vi "界面UI.vi"() -> ()   [LabVIEW 2016, in "科盛超标留样.lvlib"]
uses:
  <vilib>/Utility/miscctls.llb/LVPointTypeDef.ctl
  <vilib>/Utility/config.llb/NI_LVConfig.lvlib
  <vilib>/ptbypt/NI_PtbyPt.lvlib
panel:
  in  "超标浓度配置":bool
  in  "清除瓶记录":bool
  in  "停止流程":bool
  in  "启动流程":bool
  out "流程中":bool
  out "留样等待时间/s":dbl
  out "供样等待时间/s":dbl
  out "采样等待时间/s":dbl
  out "留样完成":bool
  out "采样完成":bool
  out "开关量3状态":T1
  out "开关量2状态":T2
  out "开关量1状态":T3
  out "元素":enum16{"open", "read", "write", "close"}(ring)
  out "供样完成":bool
  in  "返回":bool
  in  "查看记录":bool
  in  "当前解析模式":string(combo)
  in  "切换串口":bool
  out "查询系统状态":T4
  out "查询瓶记录":T5
  out "输出数组":T6(array[cluster])
  in  "留样命令":bool
  in  "供样命令":bool
  in  "触发采样":bool
  in  "查询系统状态":bool
  in  "远程取样":bool
  in  "复位指令":bool
  in  "查询瓶记录":bool
  in  "查询采样记录":bool
  in  "VISA resource name":refnum<visa-resource-name>="COM2" caption="VISA资源名称"
  in  "写入缓冲区":string
  out "读取缓冲区":string
  out "source":string
  out "通讯":bool
  # "启动顺序：先触发采样将水样取到A、B桶，然后仪器开始测试时发送供样命令此时供应到分析仪，如果超标发送留样命令，如果在默认60分钟(可设置)后都没有接受到超标留\n样指令则自动排空。按不同的采样方式发送不同的通信字符串。在一次采样未结束前不要发送下一个采样指令。"
  # "采样：将水样取到A、B桶的过程；\n供样：将水样从A、B桶供应到分析仪的过程；\n留样：将水样从A、B桶保存到采样瓶的过程。"
  # "科盛超标留样"
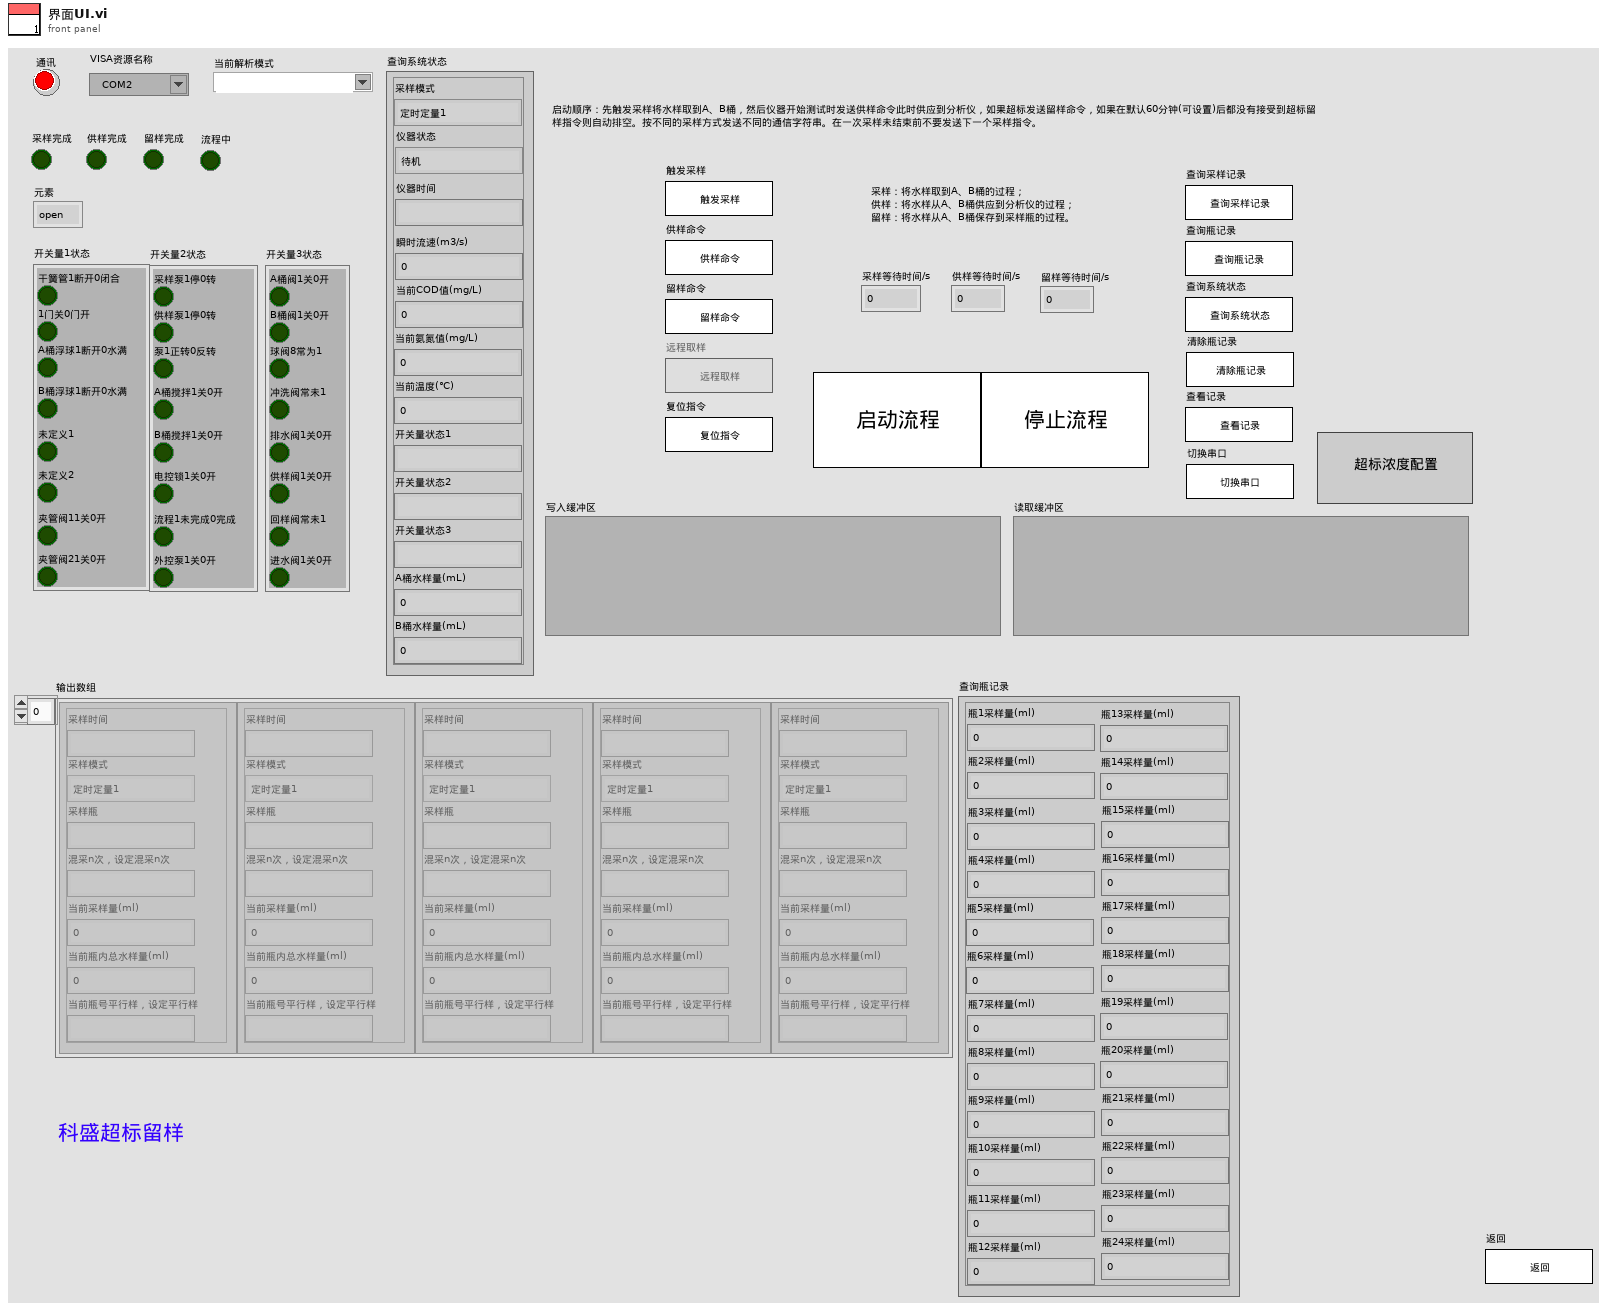
[diagram p1: front panel]
types:
  T1 = cluster{"A桶阀1关0开":bool, "B桶阀1关0开":bool, "球阀8常为1":bool, "冲洗阀常未1":bool, "排水阀1关0开":bool, "供样阀1关0开":bool, "回样阀常未1":bool, "进水阀1关0开":bool}
  T2 = cluster{"采样泵1停0转":bool, "供样泵1停0转":bool, "泵1正转0反转":bool, "A桶搅拌1关0开":bool, "B桶搅拌1关0开":bool, "电控锁1关0开":bool, "流程1未完成0完成":bool, "外控泵1关0开":bool}
  T3 = cluster{"干簧管1断开0闭合":bool, "1门关0门开":bool, "A桶浮球1断开0水满":bool, "B桶浮球1断开0水满":bool, "未定义1":bool, "未定义2":bool, "夹管阀11关0开":bool, "夹管阀21关0开":bool}
  T4 = cluster{"采样模式":enum16{"定时定量1", "定时定量2", "定流定量", "定时比例", "同步留样", "超标留样", "触发采样", "定时采样1", "定流供样", "定时采样2", "远程取样", "手动取样", "流量跟踪"}, "仪器状态":enum16{"待机", "运行中"}, "仪器时间":string, "瞬时流速(m3/s)":dbl, "当前COD值(mg/L)":dbl, "当前氨氮值(mg/L)":dbl, "当前温度(℃)":dbl, "开关量状态1":string, "开关量状态2":string, "开关量状态3":string, "A桶水样量(mL)":dbl, "B桶水样量(mL)":dbl}
  T5 = cluster{"瓶1采样量(ml)":dbl, "瓶2采样量(ml)":dbl, "瓶3采样量(ml)":dbl, "瓶4采样量(ml)":dbl, "瓶5采样量(ml)":dbl, "瓶6采样量(ml)":dbl, "瓶7采样量(ml)":dbl, "瓶8采样量(ml)":dbl, "瓶9采样量(ml)":dbl, "瓶10采样量(ml)":dbl, "瓶11采样量(ml)":dbl, "瓶12采样量(ml)":dbl, "瓶13采样量(ml)":dbl, "瓶14采样量(ml)":dbl, "瓶15采样量(ml)":dbl, "瓶16采样量(ml)":dbl, "瓶17采样量(ml)":dbl, "瓶18采样量(ml)":dbl, "瓶19采样量(ml)":dbl, "瓶20采样量(ml)":dbl, "瓶21采样量(ml)":dbl, "瓶22采样量(ml)":dbl, "瓶23采样量(ml)":dbl, "瓶24采样量(ml)":dbl}
  T6 = cluster{"采样时间":string, "采样模式":enum16{"定时定量1", "定时定量2", "定流定量", "定时比例", "同步留样", "超标留样", "触发采样", "定时采样1", "定流供样", "定时采样2", "远程取样", "手动取样", "流量跟踪"}, "采样瓶":string, "混采n次，设定混采n次":string, "当前采样量(ml)":dbl, "当前瓶内总水样量(ml)":dbl, "当前瓶号平行样，设定平行样":string}[]
  T7 = cluster{"STEP":enum16{"open", "read", "write", "close"}, "写入缓冲区":string}
  T8 = enum16{"触发采样", "供样命令", "留样命令", "远程取样", "复位指令", "查询采样记录", "查询瓶记录", "查询系统状态"}
  T9 = typedef "LVPointTypeDef.ctl" = cluster{"Horizontal":i16, "Vertical":i16}
  T10 = typedef "NI_LVConfig.lvlib/Config Data RefNum.ctl" = refnum<k1>
  T11 = cluster{"命令":string, "data":cluster{"starting address":u16, "coil values":bool[]}}
  T12 = enum8{"Enabled", "Disabled", "Disabled and Grayed Out"}
  T13 = cluster{"[0]":bool, "[1]":bool, "[2]":bool, "[3]":bool, "[4]":bool, "[5]":bool, "[6]":bool, "[7]":bool}
  T14 = cluster{"氨氮超标浓度":dbl, "总磷超标浓度":dbl, "总氮超标浓度":dbl, "CODMn超标浓度":dbl, "CODCr超标浓度":dbl}
  T15 = enum32{"Bad", "Idle", "Run top level", "Running"}
  T16 = cluster{"确定":bool, "氨氮超标浓度":dbl, "总磷超标浓度":dbl, "总氮超标浓度":dbl, "CODMn超标浓度":dbl, "CODCr超标浓度":dbl}
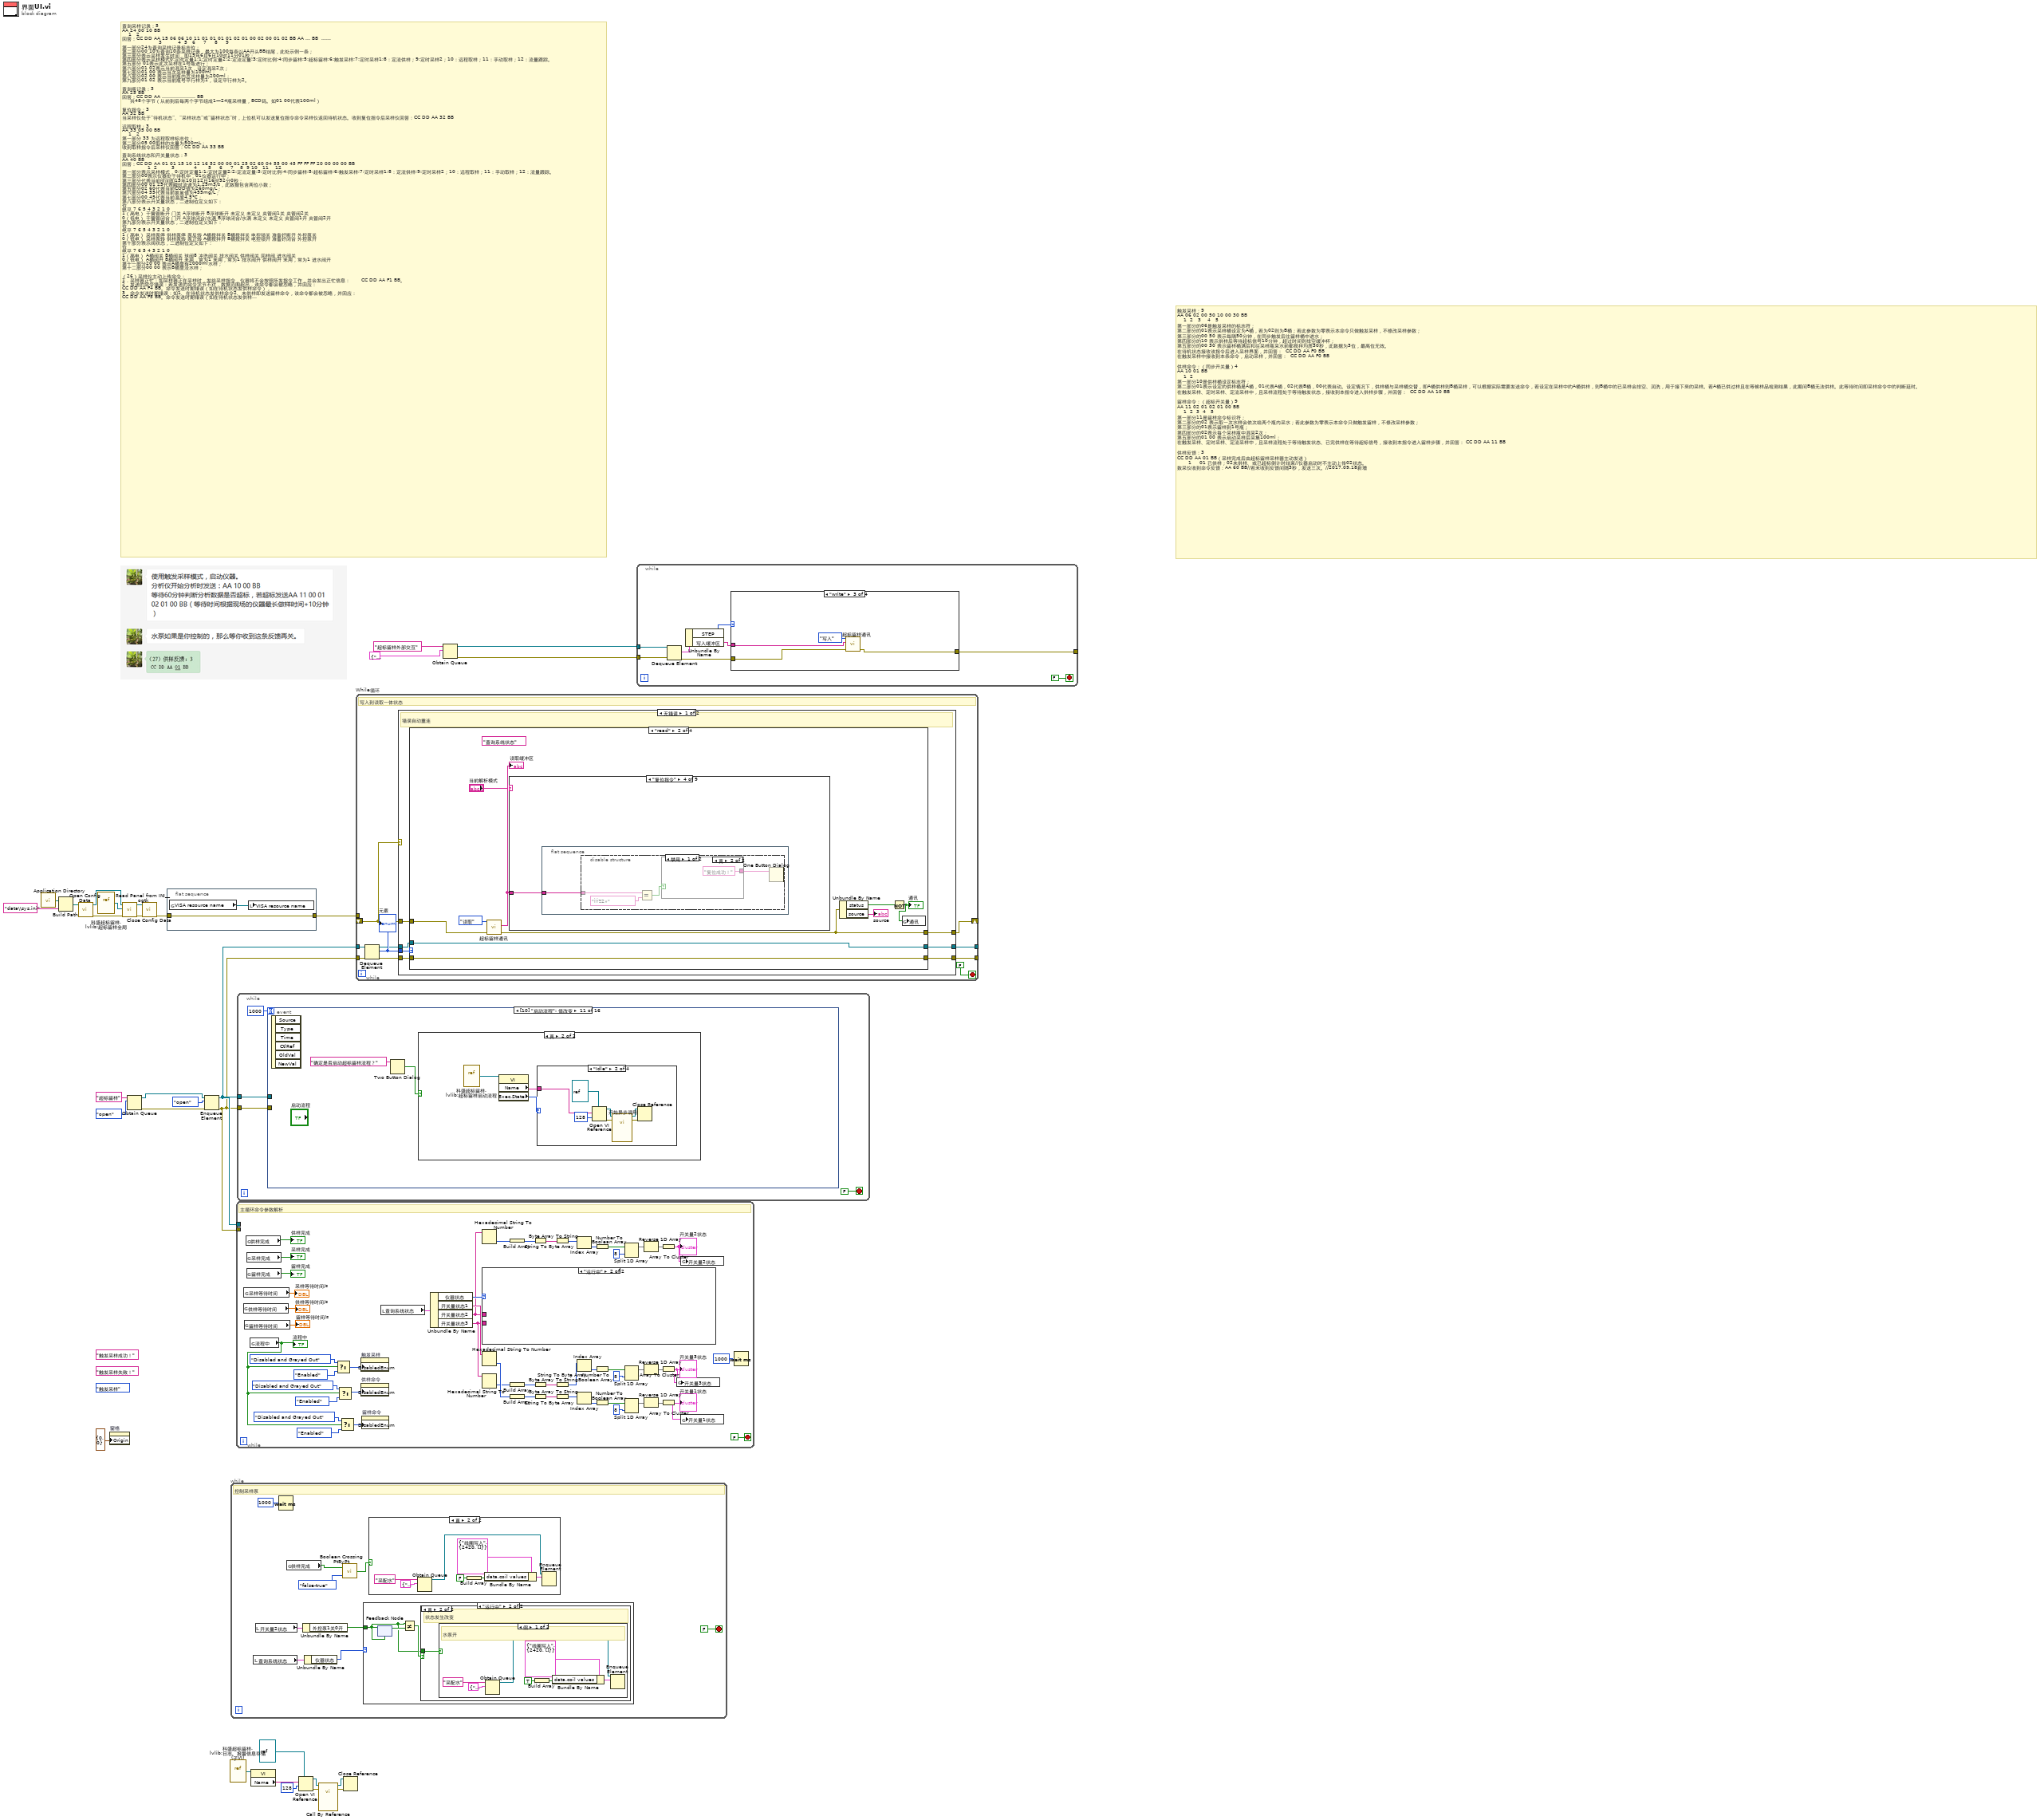
[diagram p0: block diagram]
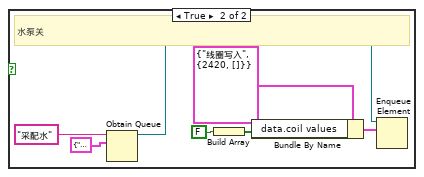
[diagram p4: hidden frame]
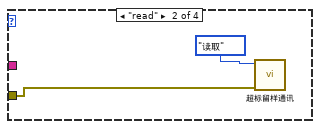
[diagram p7: hidden frame]
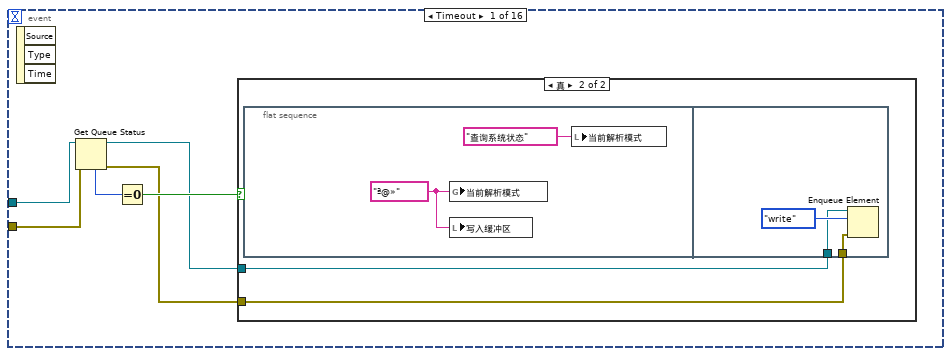
[diagram p10: hidden frame]
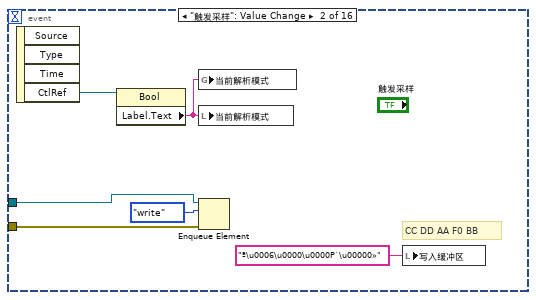
[diagram p12: hidden frame]
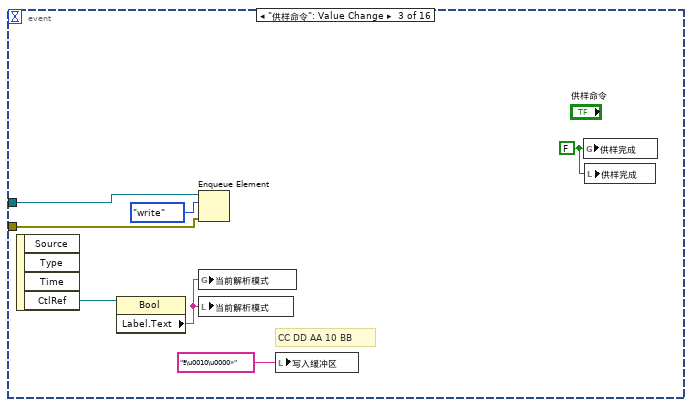
[diagram p13: hidden frame]
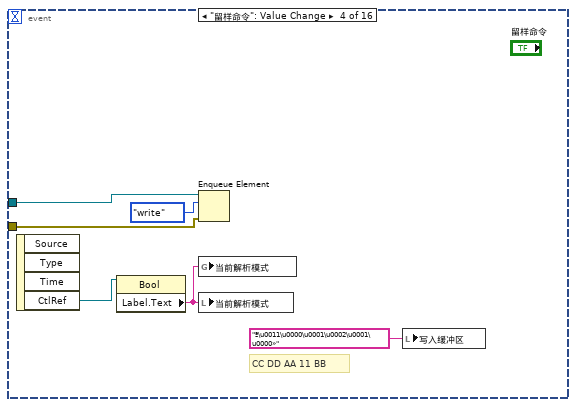
[diagram p14: hidden frame]
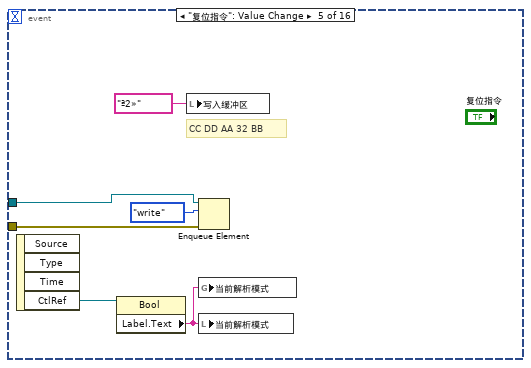
[diagram p15: hidden frame]
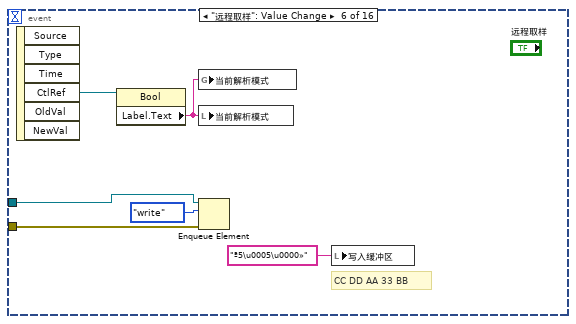
[diagram p16: hidden frame]
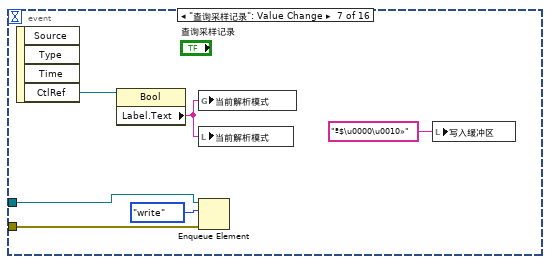
[diagram p17: hidden frame]
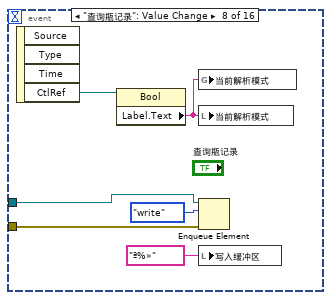
[diagram p18: hidden frame]
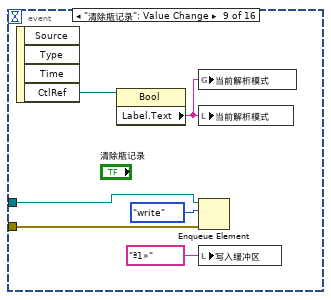
[diagram p19: hidden frame]
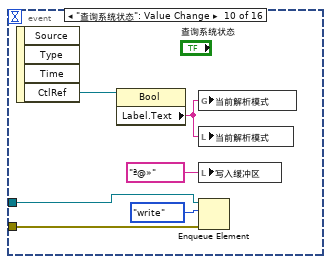
[diagram p20: hidden frame]
diagram:
  (unwired) "触发采样成功！" ("消息")
  (unwired) "触发采样失败！" ("消息")
  (unwired) T8."触发采样" ("功能输入")
  # "查询采样记录：5\nAA 24 00 10 BB\n    1   2\n回答：CC DD AA 15 06 06 10 11 01 01 01 01 02 01 00 02 00 01 02 BB AA ... BB  ......\n                       3          4  5   6     7     8     9\n第一部分24为查询采样记录标志位；\n第二部分00 10为查询10条采样记录，最大为100每条以AA开头BB结尾，此处示例一条；\n第三部分表示采样发生时间，即15年6月6日10时11分01秒；\n第四部分表示采样模式0:定时定量1;1:定时定量2;2:定流定量;3:定时比例;4:同步留样;5:超标留样;6:触发采样;7:定时采样1;8：定流供样；9:定时采样2；10：远程取样；11：手动取样；12：流量跟踪。\n第五部分 01表示此次采样在1号瓶进行；\n第六部分01 02表示当前混采1次，设定混采2次；\n第七部分01 00 表示当次采样量为100ml；\n第八部分02 00 表示当前瓶内总水样量为200ml；\n第九部分01 02 表示当前瓶号平行样为1，设定平行样为2。\n\n查询瓶记录：3\nAA 25 BB\n回答：CC DD AA ………………… BB\n     共48个字节（从前到后每两个字节组成1—24瓶采样量，BCD码。如01 00代表100ml）\n\n复位指令：3\nAA 32 BB\n当采样仪处于“待机状态”、“采样状态”或“留样状态”时，上位机可以发送复位指令命令采样仪返回待机状态。收到复位指令后采样仪回答：CC DD AA 32 BB\n\n远程取样：3\nAA 33 05 00 BB\n    1   2\n第一部分 33 为远程取样标志位；\n第二部分05 00取样的水量为500mL；\n收到取样指令后采样仪回答：CC DD AA 33 BB\n\n查询系统状态和开关量状态：3\nAA 40 BB\n回答：CC DD AA 01 01 15 10 12 16 52 00 00 01 25 02 60 04 55 00 45 FF FF FF 20 00 00 00 BB \n                1  2         3            4       5     6     7    8  9 10   11    12  \n第一部分表示采样模式，0:定时定量1;1:定时定量2;2:定流定量;3:定时比例;4:同步留样;5:超标留样;6:触发采样;7:定时采样1;8：定流供样;9:定时采样2；10：远程取样；11：手动取样；12：流量跟踪。\n第二部分00表示仪器处于待机中，01仪器运行中；\n第三部分代表当前时间即15年10月12日16时52分0秒； \n第四部分00 01 25代表瞬时流速为1.25m3/s，此数据包含两位小数；\n第五部分02 60代表当前COD值为260mg/L；\n第六部分04 55代表当前氨氮值为455mg/L；\n第七部分00 45代表当前温度4.5℃；\n第八部分表示开关量状态，二进制位定义如下：\n位\n电平\t7\t6\t5\t4\t3\t2\t1\t0\n1（高电）\t干簧管断开\t门关\tA浮球断开\tB浮球断开\t未定义\t未定义\t夹管阀1关\t夹管阀2关\n0（低电）\t干簧管闭合\t门开\tA浮球闭合/水满\tB浮球闭合/水满\t未定义\t未定义\t夹管阀1开\t夹管阀2开\n第九部分表示开关量状态，二进制位定义如下：\n位\n电平\t7\t6\t5\t4\t3\t2\t1\t0\n1（高电）\t采样泵停\t供样泵停\t泵反转\tA桶搅拌关\tB桶搅拌关\t电控锁关\t准备好断开\t外控泵关\n0（低电）\t采样泵转\t供样泵转\t泵正转\tA桶搅拌开\tB桶搅拌关\t电控锁开\t准备好闭合\t外控泵开\n第十部分表示阀状态，二进制位定义如下：\n位\n电平\t7\t6\t5\t4\t3\t2\t1\t0\n1（高电）\tA桶阀关\tB桶阀关\t球阀8\t冲洗阀关\t排水阀关\t供样阀关\t回样阀\t进水阀关\n0（低电）\tA桶阀开\tB桶阀开\t未用，常为1\t未用，常为1\t排水阀开\t供样阀开\t未用，常为1\t进水阀开\n第十一部分20 00 表示A桶里有2000ml水样；\n第十二部分00 00 表示B桶里没水样；\n\n（26）采样仪主动上传命令：\n1．采样器正忙：如采样器正在采样时，发给采样指令，仪器将不会按照所发指令工作，并会发出正忙信息：\t\t     CC DD AA F1 BB。\n2．发送的命令错误：若发送的命令字节不对，数据范围超出，该命令都会被忽略，并回应：\nCC DD AA F4 BB。命令发送时期错误（如在待机状态发供样命令），\n3．命令发送时期错误：如1、在待机状态发供样命令2、未供样即发送留样命令，该命令都会被忽略，并回应：\nCC DD AA F5 BB。命令发送时期错误（如在待机状态发供样命令），\n \t4．系统切换进入忙状态：仪器主动上传CC DD AA F6 BB。\n5．系统切换进入空闲状态：仪器主动上传CC DD AA F7 BB。"
  # "触发采样：9\nAA 06 02 00 50 10 00 30 BB\n    1  2   3    4   5         \n第一部分的06是触发采样的标志符；\n第二部分的01表示采样桶设定为A桶，若为02则为B桶；若此参数为零表示本命令只做触发采样，不修改采样参数；\n第三部分的00 50 表示每隔50分钟，在同步触发后往留样桶中进水；\n第四部分的10 表示供样后等待超标信号10分钟，超过时间则排空缓冲杯；\n第五部分的00 30 表示留样桶满后和往采样瓶采水前都搅拌均质30秒，此数据为3位，最高位无效。\n在待机状态接收该指令后进入采样界面，并回答：\t\tCC DD AA F0 BB\n在触发采样中接收到本条命令，启动采样，并回答：\t\tCC DD AA F0 BB\n\n供样命令：（同步开关量）4\nAA 10 01 BB\n    1  2  \n第一部分10是供样桶设定标志符；\n第二部分01表示设定的供样桶是A桶，01代表A桶，02代表B桶，00代表自动。设定情况下，供样桶与采样桶交替，即A桶供样则B桶采样，可以根据实际需要发送命令，若设定在采样中的A桶供样，则B桶中的已采样会排空、润洗，用于接下来的采样。若A桶已供过样且在等候样品检测结果，此期间B桶无法供样。此等待时间即采样命令中的判断延时。\n在触发采样、定时采样、定流采样中，且采样流程处于等待触发状态，接收到本指令进入供样步骤，并回答：\t\tCC DD AA 10 BB\n\n留样命令：（超标开关量）9\nAA 11 02 01 02 01 00 BB\n    1  2  3  4   5    \n第一部分11是留样命令标识符；\n第二部分的02 表示取一次水样会依次给两个瓶内采水；若此参数为零表示本命令只做触发留样，不修改采样参数；\n第三部分的01表示留样到1号瓶；\n第四部分的02表示每个采样瓶中混采2次；\n第五部分的01 00 表示启动采样后采集100ml；\n在触发采样、定时采样、定流采样中，且采样流程处于等待触发状态、已完供样在等待超标信号，接收到本指令进入留样步骤，并回答：\tCC DD AA 11 BB\n\n供样反馈：3\nCC DD AA 01 BB（采样完成后由超标留样采样器主动发送）\n  \t\t   1  \t\t\t01 已供样；02未供样、或已超标倒计时结束//仪器启动时不主动上传02状态。\n数采仪收到命令反馈：AA 60 BB//若未收到反馈间隔3秒，发送三次。//2017.09.18新增"
  n1 = call <vilib>:"Application Directory.vi"() -> ("Application Directory"=w22:path)
  n2 = Build Path(base path=w22, name or relative path="data\\sys.ini" ("名称或相对路径")) -> (appended path=w20:path)
  n3 = call <vilib>:"Open Config Data.vi"("configuration file path"=w20) -> ("error out"=w16:errorcluster, "refnum"=w19:T10)  [unwired: 8 in, 1 out]
  n4 = vi-ref "科盛超标留样.lvlib:超标留样全局.vi"() -> (w18:refnum<vi>)
  n5 = property on="窗格" class="Pane"("Origin"=T9 {"Horizontal"=0, "Vertical"=0} ("原点")) -> ()  [unwired: 2 in, 2 out]
  n6 = call <userlib>:"Read Panel from INI__ogtk.vi"("error in (no error)"=w16, "VI ref"=w18, "refnum"=w19) -> ("error out"=w15:errorcluster, "refnum out"=w17:T10)  [unwired: 7 in]
  n7 = Obtain Queue(name (unnamed)="超标留样" ("名称（未命名）"), element data type=enum16{"open", "read", "write", "close"}."open") -> (queue out=w28:refnum<queue>, error out=w27:errorcluster)  [unwired: 3 in, 1 out]
  n8 = call <vilib>:"Close Config Data.vi"("error in (no error)"=w15, "refnum"=w17) -> ("error out"=w14:errorcluster)  [unwired: 8 in, 1 out]
  n9 = flat-sequence {
    tunnel: w14 -> [w31]
    tunnel: [w31] -> w13
    frame #0 {
      n10 = global read "超标留样全局.vi" "VISA resource name"() -> (w32:refnum<visa-resource-name>)
      n11 = local write "VISA resource name"(w32) -> ()
    }
  }
  n12 = Enqueue Element(queue=w28, element=enum16{"open", "read", "write", "close"}."open", error in (no error)=w27) -> (queue out=w25:refnum<queue>, error out=w24:errorcluster)  [unwired: 1 in, 1 out]
  n13 = vi-ref "科盛超标留样.lvlib:日志、报警信息存储 (子VI).vi"() -> (w8:refnum<vi>)
  n14 = while {
    stop <- FALSE stop-if-true
    # "控制采样泵"
    n15 = local read "查询系统状态"() -> (w35:T4)
    n16 = local read "开关量2状态"() -> (w36:T2)
    n17 = Wait (ms)(milliseconds to wait=u32 1000 ("等待时间（毫秒）")) -> ()  [unwired: 1 out]
    n18 = global read "超标留样全局.vi" "供样完成"() -> (w38:bool)
    n19 = Unbundle By Name(w36) -> ("外控泵1关0开"=w33:bool)
    n20 = Unbundle By Name(w35) -> ("仪器状态"=w34:enum16{"待机", "运行中"})
    n21 = call <vilib>:"Boolean Crossing PtByPt.vi"("direction"=enum16{"either", "false-true", "true-false"}."false-true", "input"=w38) -> ("crossing"=w37:bool)  [unwired: 1 in]
    n22 = case shown="\"运行中\"" w34 {
      tunnel: w33 -> [_ w42]
      frame "待机", Default {
      }
      frame "运行中" {
        n23 = feedback-in #1(w42) -> ()
        n24 = feedback #1(w42) -> (w44:bool)
        n25 = Not Equal?(x=w42, y=w44) -> (x != y?=w43:bool)
        n26 = case shown="真" w43 {
          tunnel: w42 -> [_ w45]
          frame False {
          }
          frame True {
            # "状态发生改变"
            n27 = case shown="假" w45 {
              frame False {
                # "水泵开"
                n28 = Obtain Queue(name (unnamed)="采配水" ("名称（未命名）"), element data type=cluster{"命令":string, "数据":variant} {"命令"="", "数据"=variant}) -> (queue out=w46:refnum<queue>)  [unwired: 3 in, 2 out]
                n29 = Build Array(TRUE) -> (w49:bool[])
                n30 = Bundle By Name(cluster=T11 {"命令"="线圈写入", "data"={"starting address"=2420, "coil values"=[]}} ("元素"), "data.coil values"=w49) -> (w51:T11)
                n31 = Enqueue Element(queue=w46, element=w51) -> ()  [unwired: 2 in, 3 out]
              }
              frame True {
                # "水泵关"
                n32 = Obtain Queue(name (unnamed)="采配水" ("名称（未命名）"), element data type=cluster{"命令":string, "数据":variant} {"命令"="", "数据"=variant}) -> (queue out=w53:refnum<queue>)  [unwired: 3 in, 2 out]
                n33 = Build Array(FALSE) -> (w56:bool[])
                n34 = Bundle By Name(cluster=T11 {"命令"="线圈写入", "data"={"starting address"=2420, "coil values"=[]}} ("元素"), "data.coil values"=w56) -> (w58:T11)
                n35 = Enqueue Element(queue=w53, element=w58) -> ()  [unwired: 2 in, 3 out]
              }
            }
          }
        }
      }
    }
    n36 = case shown="真" w37 {
      frame False {
      }
      frame True {
        n37 = Obtain Queue(name (unnamed)="采配水" ("名称（未命名）"), element data type=cluster{"命令":string, "数据":variant} {"命令"="", "数据"=variant}) -> (queue out=w60:refnum<queue>)  [unwired: 3 in, 2 out]
        n38 = Build Array(FALSE) -> (w63:bool[])
        n39 = Bundle By Name(cluster=T11 {"命令"="线圈写入", "data"={"starting address"=2420, "coil values"=[]}} ("元素"), "data.coil values"=w63) -> (w65:T11)
        n40 = Enqueue Element(queue=w60, element=w65) -> ()  [unwired: 2 in, 3 out]
      }
    }
  }
  n41 = while {
    tunnel: w25 -> [_]
    tunnel: w24 -> [_]
    stop <- FALSE stop-if-true
    # "主循环命令参数解析"
    n42 = global read "超标留样全局.vi" "供样等待时间"() -> (→"供样等待时间/s":dbl)
    n43 = global read "超标留样全局.vi" "采样等待时间"() -> (→"采样等待时间/s":dbl)
    n44 = global read "超标留样全局.vi" "留样等待时间"() -> (→"留样等待时间/s":dbl)
    n45 = global read "超标留样全局.vi" "供样完成"() -> (→"供样完成":bool)
    n46 = global read "超标留样全局.vi" "采样完成"() -> (→"采样完成":bool)
    n47 = global read "超标留样全局.vi" "留样完成"() -> (→"留样完成":bool)
    n48 = global read "超标留样全局.vi" "流程中"() -> (w69:bool)
    "流程中" <- w69
    n49 = Select(t=T12."Disabled and Grayed Out" ("禁用"), s=w69, f=T12."Enabled" ("禁用")) -> (s? t:f=w76:T12)
    n50 = Select(t=T12."Disabled and Grayed Out" ("禁用"), s=w69, f=T12."Enabled" ("禁用")) -> (s? t:f=w68:T12)
    n51 = Select(t=T12."Disabled and Grayed Out" ("禁用"), s=w69, f=T12."Enabled" ("禁用")) -> (s? t:f=w67:T12)
    n52 = property on="触发采样" class="Bool"("DisabledEnum"=w76) -> ()  [unwired: 2 in, 2 out]
    n53 = property on="供样命令" class="Bool"("DisabledEnum"=w68) -> ()  [unwired: 2 in, 2 out]
    n54 = property on="留样命令" class="Bool"("DisabledEnum"=w67) -> ()  [unwired: 2 in, 2 out]
    n55 = local read "查询系统状态"() -> (w117:T4)
    n56 = Unbundle By Name(w117) -> ("仪器状态"=w116:enum16{"待机", "运行中"}, "开关量状态1"=w91:string, "开关量状态2"=w90:string, "开关量状态3"=w89:string)
    n57 = Hexadecimal String To Number(string=w90) -> (number=w94:u32)  [unwired: 2 in, 1 out]
    n58 = case shown="\"运行中\"" w116 {
      tunnel: w90 -> [_ _]
      tunnel: w89 -> [_ _]
      frame "待机", Default {
      }
      frame "运行中" {
      }
    }
    n59 = Hexadecimal String To Number(string=w91) -> (number=w97:u32)  [unwired: 2 in, 1 out]
    n60 = Hexadecimal String To Number(string=w89) -> (number=w93:u32)  [unwired: 2 in, 1 out]
    n61 = Build Array(w94) -> (w95:u32[])
    n62 = Build Array(w93) -> (w92:u32[])
    n63 = Build Array(w97) -> (w96:u32[])
    n64 = Byte Array To String(unsigned byte array=w95) -> (string=w87:string)
    n65 = Byte Array To String(unsigned byte array=w92) -> (string=w86:string)
    n66 = Byte Array To String(unsigned byte array=w96) -> (string=w88:string)
    n67 = String To Byte Array(string=w87) -> (unsigned byte array=w106:u8[])
    n68 = String To Byte Array(string=w86) -> (unsigned byte array=w105:u8[])
    n69 = String To Byte Array(string=w88) -> (unsigned byte array=w115:u8[])
    n70 = Index Array(array=w106) -> (element=w109:u8)  [unwired: 1 in]
    n71 = Index Array(array=w105) -> (element=w102:u8)  [unwired: 1 in]
    n72 = Index Array(array=w115) -> (element=w112:u8)  [unwired: 1 in]
    n73 = Number To Boolean Array(number=w109) -> (Boolean array=w110:bool[])
    n74 = Number To Boolean Array(number=w102) -> (Boolean array=w101:bool[])
    n75 = Number To Boolean Array(number=w112) -> (Boolean array=w111:bool[])
    n76 = Split 1D Array(array=w110, index=8 ("索引")) -> (first subarray=w107:bool[])  [unwired: 1 out]
    n77 = Split 1D Array(array=w101, index=8 ("索引")) -> (first subarray=w104:bool[])  [unwired: 1 out]
    n78 = Split 1D Array(array=w111, index=8 ("索引")) -> (first subarray=w114:bool[])  [unwired: 1 out]
    n79 = Reverse 1D Array(array=w107) -> (reversed array=w99:bool[])
    n80 = Reverse 1D Array(array=w104) -> (reversed array=w98:bool[])
    n81 = Reverse 1D Array(array=w114) -> (reversed array=w100:bool[])
    n82 = Array To Cluster(array=w99) -> (cluster=w83:T13)
    "开关量2状态" <- w83
    n83 = Array To Cluster(array=w98) -> (cluster=w84:T13)
    "开关量3状态" <- w84
    n84 = Array To Cluster(array=w100) -> (cluster=w85:T13)
    "开关量1状态" <- w85
    n85 = global write "超标留样全局.vi" "开关量3状态"(w84) -> ()
    n86 = global write "超标留样全局.vi" "开关量2状态"(w83) -> ()
    n87 = global write "超标留样全局.vi" "开关量1状态"(w85) -> ()
    n88 = Wait (ms)(milliseconds to wait=u32 1000 ("等待时间（毫秒）")) -> ()  [unwired: 1 out]
  }
  n89 = while {
    tunnel: w25 -> [w122]
    tunnel: w24 -> [w121]
    stop <- FALSE stop-if-true
    n90 = event shown="[10] \"启动流程\": 值改变" {
      selector: _ -> [_ _ _ _ _ _ _ _ _ _ _ _ _ _ _ _]
      dyn-events: _ -> [_ _ _ _ _ _ _ _ _ _ _ _ _ _ _ _]
      timeout: 1000 -> [_ _ _ _ _ _ _ _ _ _ _ _ _ _ _ _]
      tunnel: w122 -> [w128 w141 w147 w154 w160 w166 w172 w178 w184 w190 _ w205 w219 _ _ _]
      tunnel: w121 -> [w127 w140 w148 w153 w159 w165 w171 w177 w183 w189 _ w204 w220 _ _ _]
      event Timeout {
        n91 = event-data() -> ()  [unwired: 1 in, 3 out]
        n92 = Get Queue Status(queue=w128, error in (no error)=w127) -> (queue out=w125:refnum<queue>, error out=w124:errorcluster, # elements in queue=w129:i32)  [unwired: 1 in, 5 out]
        n93 = Equal To 0?(x=w129) -> (x = 0?=w126:bool)
        n94 = case shown="真" w126 {
          tunnel: w125 -> [_ w131]
          tunnel: w124 -> [_ w130]
          frame False {
          }
          frame True {
            n95 = flat-sequence {
              tunnel: w131 -> [w135]
              tunnel: w130 -> [w134]
              frame #0 {
                w133 = "ª@»" ("写入缓冲区")
                n96 = global write "超标留样全局.vi" "当前解析模式"(w133) -> ()
                n97 = local write "写入缓冲区"(w133) -> ()
                n98 = local write "当前解析模式"("查询系统状态" ("当前解析模式")) -> ()
              }
              frame #1 {
                n99 = Enqueue Element(queue=w135, element=enum16{"open", "read", "write", "close"}."write" ("元素"), error in (no error)=w134) -> ()  [unwired: 1 in, 3 out]
              }
            }
          }
        }
      }
      event "触发采样": Value Change {
        # "CC DD AA F0 BB"
        n100 = event-data() -> ("CtlRef"=w139:refnum<vi>)  [unwired: 1 in, 3 out]
        n101 = property class="Bool"(reference=w139) -> ("Label.Text"=w137:string)  [unwired: 1 in, 2 out]
        n102 = global write "超标留样全局.vi" "当前解析模式"(w137) -> ()
        n103 = local write "当前解析模式"(w137) -> ()
        n104 = Enqueue Element(queue=w141, element=enum16{"open", "read", "write", "close"}."write" ("元素"), error in (no error)=w140) -> ()  [unwired: 1 in, 3 out]
        n105 = local write "写入缓冲区"("ª\u0006\u0000\u0000P`\u00000»" ("写入缓冲区")) -> ()
      }
      event "供样命令": Value Change {
        w143 = FALSE ("供样完成")
        # "CC DD AA 10 BB"
        n106 = event-data() -> ("CtlRef"=w146:refnum<vi>)  [unwired: 1 in, 3 out]
        n107 = property class="Bool"(reference=w146) -> ("Label.Text"=w144:string)  [unwired: 1 in, 2 out]
        n108 = Enqueue Element(queue=w147, element=enum16{"open", "read", "write", "close"}."write" ("元素"), error in (no error)=w148) -> ()  [unwired: 1 in, 3 out]
        n109 = global write "超标留样全局.vi" "当前解析模式"(w144) -> ()
        n110 = local write "当前解析模式"(w144) -> ()
        n111 = local write "写入缓冲区"("ª\u0010\u0000»" ("写入缓冲区")) -> ()
        n112 = global write "超标留样全局.vi" "供样完成"(w143) -> ()
        n113 = local write "供样完成"(w143) -> ()
      }
      event "留样命令": Value Change {
        # "CC DD AA 11 BB"
        n114 = event-data() -> ("CtlRef"=w152:refnum<vi>)  [unwired: 1 in, 3 out]
        n115 = property class="Bool"(reference=w152) -> ("Label.Text"=w150:string)  [unwired: 1 in, 2 out]
        n116 = Enqueue Element(queue=w154, element=enum16{"open", "read", "write", "close"}."write" ("元素"), error in (no error)=w153) -> ()  [unwired: 1 in, 3 out]
        n117 = global write "超标留样全局.vi" "当前解析模式"(w150) -> ()
        n118 = local write "当前解析模式"(w150) -> ()
        n119 = local write "写入缓冲区"("ª\u0011\u0000\u0001\u0002\u0001\u0000»" ("写入缓冲区")) -> ()
      }
      event "复位指令": Value Change {
        # "CC DD AA 32 BB"
        n120 = event-data() -> ("CtlRef"=w158:refnum<vi>)  [unwired: 1 in, 3 out]
        n121 = property class="Bool"(reference=w158) -> ("Label.Text"=w156:string)  [unwired: 1 in, 2 out]
        n122 = local write "写入缓冲区"("ª2»" ("写入缓冲区")) -> ()
        n123 = Enqueue Element(queue=w160, element=enum16{"open", "read", "write", "close"}."write" ("元素"), error in (no error)=w159) -> ()  [unwired: 1 in, 3 out]
        n124 = global write "超标留样全局.vi" "当前解析模式"(w156) -> ()
        n125 = local write "当前解析模式"(w156) -> ()
      }
      event "远程取样": Value Change {
        # "CC DD AA 33 BB"
        n126 = event-data() -> ("CtlRef"=w164:refnum<vi>)  [unwired: 1 in, 5 out]
        n127 = property class="Bool"(reference=w164) -> ("Label.Text"=w162:string)  [unwired: 1 in, 2 out]
        n128 = global write "超标留样全局.vi" "当前解析模式"(w162) -> ()
        n129 = local write "当前解析模式"(w162) -> ()
        n130 = Enqueue Element(queue=w166, element=enum16{"open", "read", "write", "close"}."write" ("元素"), error in (no error)=w165) -> ()  [unwired: 1 in, 3 out]
        n131 = local write "写入缓冲区"("ª5\u0005\u0000»" ("写入缓冲区")) -> ()
      }
      event "查询采样记录": Value Change {
        n132 = event-data() -> ("CtlRef"=w170:refnum<vi>)  [unwired: 1 in, 3 out]
        n133 = property class="Bool"(reference=w170) -> ("Label.Text"=w168:string)  [unwired: 1 in, 2 out]
        n134 = global write "超标留样全局.vi" "当前解析模式"(w168) -> ()
        n135 = local write "当前解析模式"(w168) -> ()
        n136 = Enqueue Element(queue=w172, element=enum16{"open", "read", "write", "close"}."write" ("元素"), error in (no error)=w171) -> ()  [unwired: 1 in, 3 out]
        n137 = local write "写入缓冲区"("ª$\u0000\u0010»" ("写入缓冲区")) -> ()
      }
      event "查询瓶记录": Value Change {
        n138 = event-data() -> ("CtlRef"=w176:refnum<vi>)  [unwired: 1 in, 3 out]
        n139 = property class="Bool"(reference=w176) -> ("Label.Text"=w174:string)  [unwired: 1 in, 2 out]
        n140 = global write "超标留样全局.vi" "当前解析模式"(w174) -> ()
        n141 = local write "当前解析模式"(w174) -> ()
        n142 = Enqueue Element(queue=w178, element=enum16{"open", "read", "write", "close"}."write" ("元素"), error in (no error)=w177) -> ()  [unwired: 1 in, 3 out]
        n143 = local write "写入缓冲区"("ª%»" ("写入缓冲区")) -> ()
      }
      event "清除瓶记录": Value Change {
        n144 = event-data() -> ("CtlRef"=w182:refnum<vi>)  [unwired: 1 in, 3 out]
        n145 = property class="Bool"(reference=w182) -> ("Label.Text"=w180:string)  [unwired: 1 in, 2 out]
        n146 = global write "超标留样全局.vi" "当前解析模式"(w180) -> ()
        n147 = local write "当前解析模式"(w180) -> ()
        n148 = Enqueue Element(queue=w184, element=enum16{"open", "read", "write", "close"}."write" ("元素"), error in (no error)=w183) -> ()  [unwired: 1 in, 3 out]
        n149 = local write "写入缓冲区"("ª1»" ("写入缓冲区")) -> ()
      }
      event "查询系统状态": Value Change {
        n150 = event-data() -> ("CtlRef"=w188:refnum<vi>)  [unwired: 1 in, 3 out]
        n151 = property class="Bool"(reference=w188) -> ("Label.Text"=w186:string)  [unwired: 1 in, 2 out]
        n152 = global write "超标留样全局.vi" "当前解析模式"(w186) -> ()
        n153 = local write "当前解析模式"(w186) -> ()
        n154 = local write "写入缓冲区"("ª@»" ("写入缓冲区")) -> ()
        n155 = Enqueue Element(queue=w190, element=enum16{"open", "read", "write", "close"}."write" ("元素"), error in (no error)=w189) -> ()  [unwired: 1 in, 3 out]
      }
      event "启动流程": Value Change {
        n156 = event-data() -> ()  [unwired: 1 in, 6 out]
        n157 = Two Button Dialog(message="确定是否启动超标留样流程？" ("消息")) -> (T button?=w192:bool)  [unwired: 2 in]
        n158 = case shown="真" w192 {
          frame False {
          }
          frame True {
            n159 = vi-ref "科盛超标留样.lvlib:超标留样启动流程.vi"() -> (w194:refnum<vi>)
            n160 = property class="VI"(reference=w194) -> ("Name"=w195:string, "Exec.State"=w196:T15)  [unwired: 1 in, 2 out]
            n161 = case shown="\"Idle\"" w196 {
              tunnel: w195 -> [_ w199 _ _]
              frame "Bad", Default {
              }
              frame "Idle" {
                n162 = Open VI Reference(type specifier VI Refnum (for type only)=refnum<vi> refnum ("类型说明符VI引用句柄（仅用于类型）"), vi path=w199, options=128 ("选项")) -> (vi reference=w203:refnum<vi>, error out=w198:errorcluster)  [unwired: 3 in]
                n163 = call-by-ref "开始异步调用"(reference=w203, error in=w198) -> (reference out=w202:refnum<vi>, error out=w197:errorcluster)  [unwired: 12 in]
                n164 = Close Reference(reference=w202, error in (no error)=w197) -> ()  [unwired: 1 out]
              }
              frame "Run top level" {
              }
              frame "Running" {
              }
            }
          }
        }
      }
      event "停止流程": Value Change {
        n165 = event-data() -> ()  [unwired: 1 in, 6 out]
        n166 = Two Button Dialog(message="确定是否停止超标留样流程？" ("消息")) -> (T button?=w206:bool)  [unwired: 2 in]
        n167 = case shown="真" w206 {
          tunnel: w205 -> [_ w209]
          tunnel: w204 -> [_ w208]
          frame False {
          }
          frame True {
            n168 = Obtain Notifier(name (unnamed)="超标留样流程" ("名称（未命名）"), notification data type=FALSE ("采样完成")) -> (notifier out=w216:refnum<notifier>, error out=w215:errorcluster)  [unwired: 2 in, 1 out]
            n169 = Send Notification(notification=TRUE ("通知"), notifier=w216, error in (no error)=w215) -> (notifier out=w213:refnum<notifier>, error out=w212:errorcluster)
            n170 = Enqueue Element(queue=w209, element=enum16{"open", "read", "write", "close"}."write" ("元素"), error in (no error)=w208) -> ()  [unwired: 1 in, 3 out]
            n171 = local write "写入缓冲区"("ª2»" ("写入缓冲区")) -> ()
            n172 = Release Notifier(notifier=w213, error in (no error)=w212) -> ()  [unwired: 1 in, 3 out]
          }
        }
      }
      event "切换串口": Value Change {
        n173 = flat-sequence {
          frame #0 {
            n174 = local read "VISA resource name"() -> (w222:refnum<visa-resource-name>)
            n175 = global write "超标留样全局.vi" "VISA resource name"(w222) -> ()
          }
          frame #1 {
            n176 = call <vilib>:"Application Directory.vi"() -> ("Application Directory"=w224:path)
            n177 = Build Path(base path=w224, name or relative path="data\\sys.ini" ("名称或相对路径")) -> (appended path=w225:path)
            n178 = call <vilib>:"Open Config Data.vi"("configuration file path"=w225) -> ("error out"=w229:errorcluster, "refnum"=w226:T10)  [unwired: 8 in, 1 out]
            n179 = vi-ref "科盛超标留样.lvlib:超标留样全局.vi"() -> (w227:refnum<vi>)
            n180 = call <userlib>:"Write Panel to INI__ogtk.vi"("error in (no error)"=w229, "VI ref"=w227, "refnum"=w226) -> ("error out"=w230:errorcluster, "refnum out"=w228:T10)  [unwired: 7 in]
            n181 = call <vilib>:"Close Config Data.vi"("error in (no error)"=w230, "refnum"=w228) -> ("error out"=w235:errorcluster, "file path"=w236:path)  [unwired: 8 in]
            n182 = Open/Create/Replace File(file path (use dialog)=w236, error in=w235) -> (refnum out=w232:refnum<file>, error out=w231:errorcluster)  [unwired: 4 in, 1 out]
            n183 = Flush File(refnum=w232, error in=w231) -> (refnum out=w233:refnum<file>, error out=w234:errorcluster)
            n184 = Close File(refnum=w233, error in=w234) -> ()  [unwired: 2 out]
          }
        }
        n185 = event-data() -> ()  [unwired: 1 in, 6 out]
        n186 = Enqueue Element(queue=w219, element=enum16{"open", "read", "write", "close"}."close" ("元素"), error in (no error)=w220) -> ()  [unwired: 1 in, 3 out]
      }
      event "超标浓度配置": Value Change {
        n187 = event-data() -> ()  [unwired: 1 in, 6 out]
        n188 = global read "超标留样全局.vi" "CODMn超标浓度"() -> (w246:dbl)
        n189 = global read "超标留样全局.vi" "CODCr超标浓度"() -> (w245:dbl)
        n190 = global read "超标留样全局.vi" "总氮超标浓度"() -> (w247:dbl)
        n191 = global read "超标留样全局.vi" "氨氮超标浓度"() -> (w248:dbl)
        n192 = global read "超标留样全局.vi" "总磷超标浓度"() -> (w249:dbl)
        n193 = Bundle By Name(cluster=T14 {"氨氮超标浓度"=0.0, "总磷超标浓度"=0.0, "总氮超标浓度"=0.0, "CODMn超标浓度"=0.0, "CODCr超标浓度"=0.0} ("输入"), "氨氮超标浓度"=w248, "总磷超标浓度"=w249, "总氮超标浓度"=w247, "CODMn超标浓度"=w246, "CODCr超标浓度"=w245) -> (w244:T14)
        n194 = call "超标浓度设置.vi"("输入"=w244) -> ("输出"=w243:T16)  [unwired: 10 in]
        n195 = Unbundle By Name(w243) -> ("确定"=w242:bool, "氨氮超标浓度"=w241:dbl, "总磷超标浓度"=w240:dbl, "总氮超标浓度"=w239:dbl, "CODMn超标浓度"=w238:dbl, "CODCr超标浓度"=w237:dbl)
        n196 = case shown="真" w242 {
          tunnel: w241 -> [_ w255]
          tunnel: w240 -> [_ w254]
          tunnel: w239 -> [_ w253]
          tunnel: w238 -> [_ w252]
          tunnel: w237 -> [_ w251]
          frame False {
          }
          frame True {
            n197 = flat-sequence {
              tunnel: w255 -> [w260]
              tunnel: w254 -> [w259]
              tunnel: w253 -> [w258]
              tunnel: w252 -> [w257]
              tunnel: w251 -> [w256]
              frame #0 {
                n198 = global write "超标留样全局.vi" "CODMn超标浓度"(w257) -> ()
                n199 = global write "超标留样全局.vi" "CODCr超标浓度"(w256) -> ()
                n200 = global write "超标留样全局.vi" "总氮超标浓度"(w258) -> ()
                n201 = global write "超标留样全局.vi" "氨氮超标浓度"(w260) -> ()
                n202 = global write "超标留样全局.vi" "总磷超标浓度"(w259) -> ()
              }
              frame #1 {
                n203 = call <vilib>:"Application Directory.vi"() -> ("Application Directory"=w262:path)
                n204 = Build Path(base path=w262, name or relative path="data\\sys.ini" ("名称或相对路径")) -> (appended path=w263:path)
                n205 = call <vilib>:"Open Config Data.vi"("configuration file path"=w263) -> ("error out"=w267:errorcluster, "refnum"=w264:T10)  [unwired: 8 in, 1 out]
                n206 = vi-ref "科盛超标留样.lvlib:超标留样全局.vi"() -> (w265:refnum<vi>)
                n207 = call <userlib>:"Write Panel to INI__ogtk.vi"("error in (no error)"=w267, "VI ref"=w265, "refnum"=w264) -> ("error out"=w268:errorcluster, "refnum out"=w266:T10)  [unwired: 7 in]
                n208 = call <vilib>:"Close Config Data.vi"("error in (no error)"=w268, "refnum"=w266) -> ("error out"=w273:errorcluster, "file path"=w274:path)  [unwired: 8 in]
                n209 = Open/Create/Replace File(file path (use dialog)=w274, error in=w273) -> (refnum out=w270:refnum<file>, error out=w269:errorcluster)  [unwired: 4 in, 1 out]
                n210 = Flush File(refnum=w270, error in=w269) -> (refnum out=w271:refnum<file>, error out=w272:errorcluster)
                n211 = Close File(refnum=w271, error in=w272) -> ()  [unwired: 2 out]
              }
            }
          }
        }
      }
      event "查看记录": Value Change {
        n212 = event-data() -> ()  [unwired: 1 in, 6 out]
        n213 = property on="窗格" class="Pane"("Origin"=T9 {"Horizontal"=0, "Vertical"=628} ("原点")) -> ()  [unwired: 2 in, 2 out]
      }
      event "返回": Value Change {
        n214 = event-data() -> ()  [unwired: 1 in, 6 out]
        n215 = property on="窗格" class="Pane"("Origin"=T9 {"Horizontal"=0, "Vertical"=0} ("原点")) -> ()  [unwired: 2 in, 2 out]
      }
    }
  }
  n216 = property class="VI"(reference=w8) -> ("Name"=w7:string)  [unwired: 1 in, 2 out]
  n217 = Open VI Reference(type specifier VI Refnum (for type only)=refnum<vi> refnum ("类型说明符VI引用句柄（仅用于类型）"), vi path=w7, options=128 ("选项")) -> (vi reference=w4:refnum<vi>, error out=w1:errorcluster)  [unwired: 3 in]
  n218 = call-by-ref "?"(reference=w4, error in=w1) -> (reference out=w3:refnum<vi>, error out=w2:errorcluster)  [unwired: 12 in]
  n219 = Close Reference(reference=w3, error in (no error)=w2) -> ()  [unwired: 1 out]
  n220 = while "While循环" {
    tunnel: w25 -> [w285]
    tunnel: w24 -> [w284]
    tunnel: [w280] -> _
    tunnel: [w279] -> _
    shift-right: [w277] -> _
    shift-left: _ -> [w278]
    tunnel: w13 -> [_]
    stop <- FALSE stop-if-true
    # "写入到读取一体状态"
    n221 = Dequeue Element(queue=w285, error in (no error)=w284) -> (queue out=w282:refnum<queue>, element=w283:enum16{"open", "read", "write", "close"}, error out=w281:errorcluster)  [unwired: 1 in, 1 out]
    "元素" <- w283
    n222 = case shown="无错误" w278 {
      tunnel: w283 -> [w293 _]
      tunnel: w282 -> [w292 w401]
      tunnel: w281 -> [w291 w400]
      tunnel: [w290 w394] -> w280
      tunnel: [w289 w393] -> w279
      tunnel: w278 -> [w288 w396]
      tunnel: [w287 w395] -> w277
      frame No Error {
        # "错误自动重连"
        n223 = case shown="\"read\"" w293 {
          tunnel: [w294 w300 w375 w389] -> w287
          tunnel: w292 -> [w297 w306 w382 w388]
          tunnel: w291 -> [w296 w305 w381 w387]
          tunnel: [w297 w306 w380 w385] -> w290
          tunnel: [w296 w305 w379 w384] -> w289
          tunnel: w288 -> [_ w308 w378 w391]
          frame "open", Default {
            (unwired) refnum<visa-resource-name> "COM2" ("VISA resource name")
            n224 = global write "超标留样全局.vi" "VISA resource name"("VISA resource name") -> ()
            n225 = call "超标留样通讯.vi"("VISA resource name"="VISA resource name", "功能输入"=enum16{"打开串口", "写入", "读取", "关闭串口"}."打开串口") -> ("error out"=w294:errorcluster)  [unwired: 7 in, 2 out]
          }
          frame "read" {
            (unwired) "查询系统状态" ("当前解析模式")
            n226 = call "超标留样通讯.vi"("error in (no error)"=w308, "功能输入"=enum16{"打开串口", "写入", "读取", "关闭串口"}."读取") -> ("error out"=w300:errorcluster, "读取缓冲区"=w304:string)  [unwired: 7 in, 1 out]
            "读取缓冲区" <- w304
            n227 = case shown="\"复位指令\"" "当前解析模式" {
              tunnel: w304 -> [w309 w317 w325 w333 w341 w348 w354 w360 w367]
              frame "触发采样" {
                n228 = flat-sequence {
                  tunnel: w309 -> [w310]
                  frame #0 {
                    n229 = disable-structure shown="禁用" {
                      disable-tunnel: w310 -> [w314 _]
                      frame Disabled {
                        n230 = Equal?(x=w314, y="ÌÝªð»") -> (x = y?=w312:bool)
                        n231 = case shown="真" w312 {
                          tunnel: ["触发采样失败！" ("消息") "触发采样成功！" ("消息")] -> w311
                          frame False {
                          }
                          frame True {
                          }
                        }
                        n232 = One Button Dialog(message=w311) -> ()  [unwired: 1 in, 1 out]
                      }
                      frame Enabled {
                      }
                    }
                  }
                }
              }
              frame "供样命令" {
                n233 = flat-sequence {
                  tunnel: w317 -> [w318]
                  frame #0 {
                    n234 = disable-structure shown="禁用" {
                      disable-tunnel: w318 -> [w322 _]
                      frame Disabled {
                        n235 = Equal?(x=w322, y="ÌÝª\u0010»") -> (x = y?=w320:bool)
                        n236 = case shown="真" w320 {
                          tunnel: ["供样失败！" ("消息") "供样成功！" ("消息")] -> w319
                          frame False {
                          }
                          frame True {
                          }
                        }
                        n237 = One Button Dialog(message=w319) -> ()  [unwired: 1 in, 1 out]
                      }
                      frame Enabled {
                      }
                    }
                  }
                }
              }
              frame "留样命令", Default {
                n238 = flat-sequence {
                  tunnel: w325 -> [w326]
                  frame #0 {
                    n239 = disable-structure shown="禁用" {
                      disable-tunnel: w326 -> [w330 _]
                      frame Disabled {
                        n240 = Equal?(x=w330, y="ÌÝª\u0011»") -> (x = y?=w328:bool)
                        n241 = case shown="真" w328 {
                          tunnel: ["留样失败！" ("消息") "留样成功！" ("消息")] -> w327
                          frame False {
                          }
                          frame True {
                          }
                        }
                        n242 = One Button Dialog(message=w327) -> ()  [unwired: 1 in, 1 out]
                      }
                      frame Enabled {
                      }
                    }
                  }
                }
              }
              frame "复位指令" {
                n243 = flat-sequence {
                  tunnel: w333 -> [w334]
                  frame #0 {
                    n244 = disable-structure shown="禁用" {
                      disable-tunnel: w334 -> [w338 _]
                      frame Disabled {
                        n245 = Equal?(x=w338, y="ÌÝª2»") -> (x = y?=w336:bool)
                        n246 = case shown="真" w336 {
                          tunnel: ["复位失败！" ("消息") "复位成功！" ("消息")] -> w335
                          frame False {
                          }
                          frame True {
                          }
                        }
                        n247 = One Button Dialog(message=w335) -> ()  [unwired: 1 in, 1 out]
                      }
                      frame Enabled {
                      }
                    }
                  }
                }
              }
              frame "远程取样" {
                n248 = flat-sequence {
                  tunnel: w341 -> [w345]
                  frame #0 {
                    n249 = Equal?(x=w345, y="ÌÝª3»") -> (x = y?=w343:bool)
                    n250 = case shown="假" w343 {
                      tunnel: ["远程取样失败！" ("消息") "远程取样成功！" ("消息")] -> w342
                      frame False {
                      }
                      frame True {
                      }
                    }
                    n251 = One Button Dialog(message=w342) -> ()  [unwired: 1 in, 1 out]
                  }
                }
              }
              frame "查询采样记录" {
                n252 = flat-sequence {
                  tunnel: w348 -> [w353]
                  frame #0 {
                    n253 = call "科盛查询命令解析.vi"("解析参数选择"=enum16{"查询采样记录", "查询瓶记录", "查询系统状态"}."查询采样记录", "命令输入"=w353) -> ("Variant"=w351:variant)  [unwired: 9 in]
                    n254 = Variant To Data(type=T6 [] ("输出数组"), Variant=w351) -> (data=→"输出数组":T6)  [unwired: 1 in, 1 out]
                  }
                }
              }
              frame "查询瓶记录" {
                n255 = flat-sequence {
                  tunnel: w354 -> [w359]
                  frame #0 {
                    n256 = call "科盛查询命令解析.vi"("解析参数选择"=enum16{"查询采样记录", "查询瓶记录", "查询系统状态"}."查询瓶记录", "命令输入"=w359) -> ("Variant"=w357:variant)  [unwired: 9 in]
                    n257 = Variant To Data(type=T5 {"瓶1采样量(ml)"=0.0, "瓶2采样量(ml)"=0.0, "瓶3采样量(ml)"=0.0, "瓶4采样量(ml)"=0.0, "瓶5采样量(ml)"=0.0, "瓶6采样量(ml)"=0.0, "瓶7采样量(ml)"=0.0, "瓶8采样量(ml)"=0.0, "瓶9采样量(ml)"=0.0, "瓶10采样量(ml)"=0.0, "瓶11采样量(ml)"=0.0, "瓶12采样量(ml)"=0.0, "瓶13采样量(ml)"=0.0, "瓶14采样量(ml)"=0.0, "瓶15采样量(ml)"=0.0, "瓶16采样量(ml)"=0.0, "瓶17采样量(ml)"=0.0, "瓶18采样量(ml)"=0.0, "瓶19采样量(ml)"=0.0, "瓶20采样量(ml)"=0.0, "瓶21采样量(ml)"=0.0, "瓶22采样量(ml)"=0.0, "瓶23采样量(ml)"=0.0, "瓶24采样量(ml)"=0.0} ("查询瓶记录"), Variant=w357) -> (data=→"查询瓶记录":T5)  [unwired: 1 in, 1 out]
                  }
                }
              }
              frame "清除瓶记录" {
                n258 = flat-sequence {
                  tunnel: w360 -> [w364]
                  frame #0 {
                    n259 = Equal?(x=w364, y="ÌÝª1»") -> (x = y?=w362:bool)
                    n260 = case shown="假" w362 {
                      tunnel: ["清除失败！" ("消息") "清除成功！" ("消息")] -> w361
                      frame False {
                      }
                      frame True {
                      }
                    }
                    n261 = One Button Dialog(message=w361) -> ()  [unwired: 1 in, 1 out]
                  }
                }
              }
              frame "查询系统状态" {
                n262 = flat-sequence {
                  tunnel: w367 -> [w368]
                  frame #0 {
                    n263 = case shown="\"假\", 默认" w368 {
                      tunnel: w368 -> [w371 _]
                      frame "假", Default {
                        n264 = call "科盛查询命令解析.vi"("解析参数选择"=enum16{"查询采样记录", "查询瓶记录", "查询系统状态"}."查询系统状态", "命令输入"=w371) -> ("Variant"=w373:variant)  [unwired: 9 in]
                        n265 = Variant To Data(type=T4 {"采样模式"=enum."定时定量1", "仪器状态"=enum."待机", "仪器时间"="", "瞬时流速(m3/s)"=0.0, "当前COD值(mg/L)"=0.0, "当前氨氮值(mg/L)"=0.0, "当前温度(℃)"=0.0, "开关量状态1"="", "开关量状态2"="", "开关量状态3"="", "A桶水样量(mL)"=0.0, "B桶水样量(mL)"=0.0} ("查询系统状态"), Variant=w373) -> (data=w370:T4)  [unwired: 1 in, 1 out]
                        "查询系统状态" <- w370
                        n266 = global write "超标留样全局.vi" "查询系统状态"(w370) -> ()
                      }
                      frame "" {
                      }
                    }
                    n267 = Equal?(x=w368, y="ÌÝª\u0001»") -> ()  [unwired: 1 out]
                  }
                }
              }
            }
            n268 = Unbundle By Name(w300) -> ("status"=w302:bool, "source"=→"source":string)
            n269 = Not(x=w302) -> (.not. x?=w299:bool)
            "通讯" <- w299
            n270 = global write "超标留样全局.vi" "通讯"(w299) -> ()
          }
          frame "write" {
            n271 = Enqueue Element(queue=w382, element=enum16{"open", "read", "write", "close"}."read" ("元素"), error in (no error)=w381) -> (queue out=w380:refnum<queue>, error out=w379:errorcluster)  [unwired: 1 in, 1 out]
            n272 = call "超标留样通讯.vi"("error in (no error)"=w378, "写入缓冲区"="写入缓冲区", "功能输入"=enum16{"打开串口", "写入", "读取", "关闭串口"}."写入") -> ("error out"=w375:errorcluster)  [unwired: 6 in, 2 out]
          }
          frame "close" {
            n273 = Enqueue Element(queue=w388, element=enum16{"open", "read", "write", "close"}."open" ("元素"), error in (no error)=w387) -> (queue out=w385:refnum<queue>, error out=w384:errorcluster)  [unwired: 1 in, 1 out]
            n274 = call "超标留样通讯.vi"("error in (no error)"=w391, "功能输入"=enum16{"打开串口", "写入", "读取", "关闭串口"}."关闭串口") -> ("error out"=w389:errorcluster)  [unwired: 7 in, 2 out]
          }
        }
      }
      frame Error {
        n275 = Flush Queue(queue=w401, error in (no error)=w400) -> (queue out=w399:refnum<queue>, error out=w398:errorcluster)  [unwired: 1 out]
        n276 = call <vilib>:"Clear Errors.vi"("error in (no error)"=w396) -> ("error out"=w395:errorcluster)  [unwired: 5 in, 1 out]
        n277 = Enqueue Element(queue=w399, element=enum16{"open", "read", "write", "close"}."close" ("元素"), error in (no error)=w398) -> (queue out=w394:refnum<queue>, error out=w393:errorcluster)  [unwired: 1 in, 1 out]
        n278 = Wait (ms)(milliseconds to wait=u32 2000 ("等待时间（毫秒）")) -> ()  [unwired: 1 out]
      }
    }
  }
  n279 = Obtain Queue(name (unnamed)="超标留样外部交互" ("名称（未命名）"), element data type=T7 {"STEP"=enum."write", "写入缓冲区"="ª\u0006\u0000\u0000P`\u00000»"}) -> (queue out=w10:refnum<queue>, error out=w9:errorcluster)  [unwired: 3 in, 1 out]
  n280 = while {
    tunnel: w10 -> [w408]
    tunnel: w9 -> [w407]
    tunnel: [w402] -> _
    stop <- FALSE stop-if-true
    n281 = Dequeue Element(queue=w408, error in (no error)=w407) -> (element=w406:T7, error out=w404:errorcluster)  [unwired: 1 in, 2 out]
    n282 = Unbundle By Name(w406) -> ("STEP"=w405:enum16{"open", "read", "write", "close"}, "写入缓冲区"=w403:string)
    n283 = case shown="\"write\"" w405 {
      tunnel: w404 -> [_ w410 w414 _]
      tunnel: w403 -> [_ _ w413 _]
      tunnel: [_ _ w412 _] -> w402
      frame "open", Default {
      }
      frame "read" {
        n284 = call "超标留样通讯.vi"("error in (no error)"=w410, "功能输入"=enum16{"打开串口", "写入", "读取", "关闭串口"}."读取") -> ()  [unwired: 7 in, 3 out]
      }
      frame "write" {
        n285 = call "超标留样通讯.vi"("error in (no error)"=w414, "写入缓冲区"=w413, "功能输入"=enum16{"打开串口", "写入", "读取", "关闭串口"}."写入") -> ("error out"=w412:errorcluster)  [unwired: 6 in, 2 out]
      }
      frame "close" {
      }
    }
  }
